vi "Param_Sys.vi"() -> ()   [LabVIEW 2020]
panel:
  out "Vrange":dbl
  out "DCIR timeout":dbl
  out "Timeouttest":dbl
  out "Baud Rate":dbl
  out "SOC70Vmax":dbl
  out "SOC70Vmin":dbl
  out "SOC30Vmax":dbl
  out "SOC30Vmin":dbl
  out "Poste":string
  out "RefFichConf":string
  out "VISA OUT":T1={"Hitech"="", "multi"="", "5520"="", "3562"="", "TakTak"="Arduino Uno"}
  out "ModeAuto?":bool
  out "Lower limite value":dbl
  # "Hioki 5520"
  # "Hioki BT3562"
  # "DCIR"
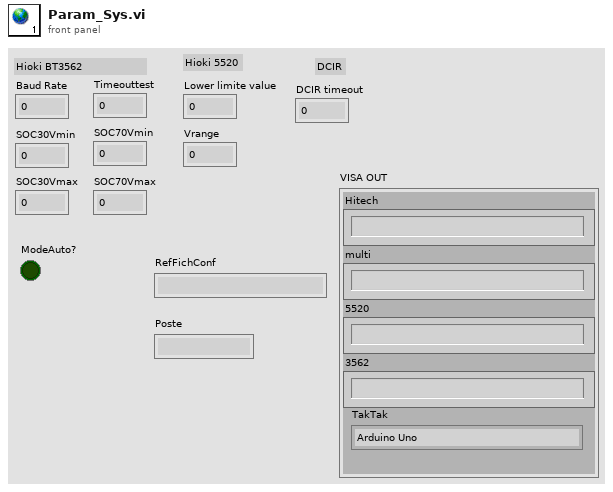
[diagram p1: front panel]
types:
  T1 = cluster{"Hitech":string, "multi":string, "5520":string, "3562":string, "TakTak":string}
diagram:
